vi "Teleop.vi"(10 "Match Info":T1={"Autonomous Elapsed Seconds"=0.0, "TeleOp Elapsed Seconds"=0.0, "Disabled Elapsed Seconds"=0.0, "Visited Autonomous"=FALSE, "Visited TeleOp"=FALSE, "Visited Disabled"=FALSE, "Autonomous Settings"={"Autonomous Style"=enum."Independent", "VI Refnum"=refnum}}, 11 "Call Context":T2) -> ()   [LabVIEW 2015]
doc: "This VI is called for each TeleOp packet received from the DS where the robot is not disabled. It is often used to read from the joysticks and update I/O or to update setpoints for timed control loops. It should complete and return within 20 milliseconds or it may miss DS packets."
uses:
  <vilib>/Rock Robotics/WPI/DriverStation/WPI_DriverStationDerivedRobotMode.ctl
  <vilib>/Rock Robotics/WPI/DriverStation/WPI_DriverStationMatch Info.ctl
  <vilib>/Rock Robotics/WPI/Solenoid/WPI_SolenoidValue.ctl
  <vilib>/Rock Robotics/Network Tables/NT Read Boolean.vi
  <vilib>/Rock Robotics/Network Tables/NT Read Number.vi
  <vilib>/Rock Robotics/WPI/Utilities/WPI_GetSetVariantRefNum.vi
  <vilib>/Rock Robotics/WPI/Solenoid/WPI_SolenoidSetEnum.vi
  <vilib>/addons/control/pid/pid.llb/PID (DBL).vi
  <vilib>/addons/control/pid/NI_PID_pid.lvlib
panel:
  in  "Numeric":dbl
  out "Encodeur gauche min":dbl
  out "Encodeur gauche max":dbl
  out "Encodeur droit max":dbl
  out "Encodeur droit min":dbl
  out "Sample Slider 0":dbl(slide) scale=0.0..5.0
  out "Sample Boolean 1":bool
  out "Sample Boolean 0":bool
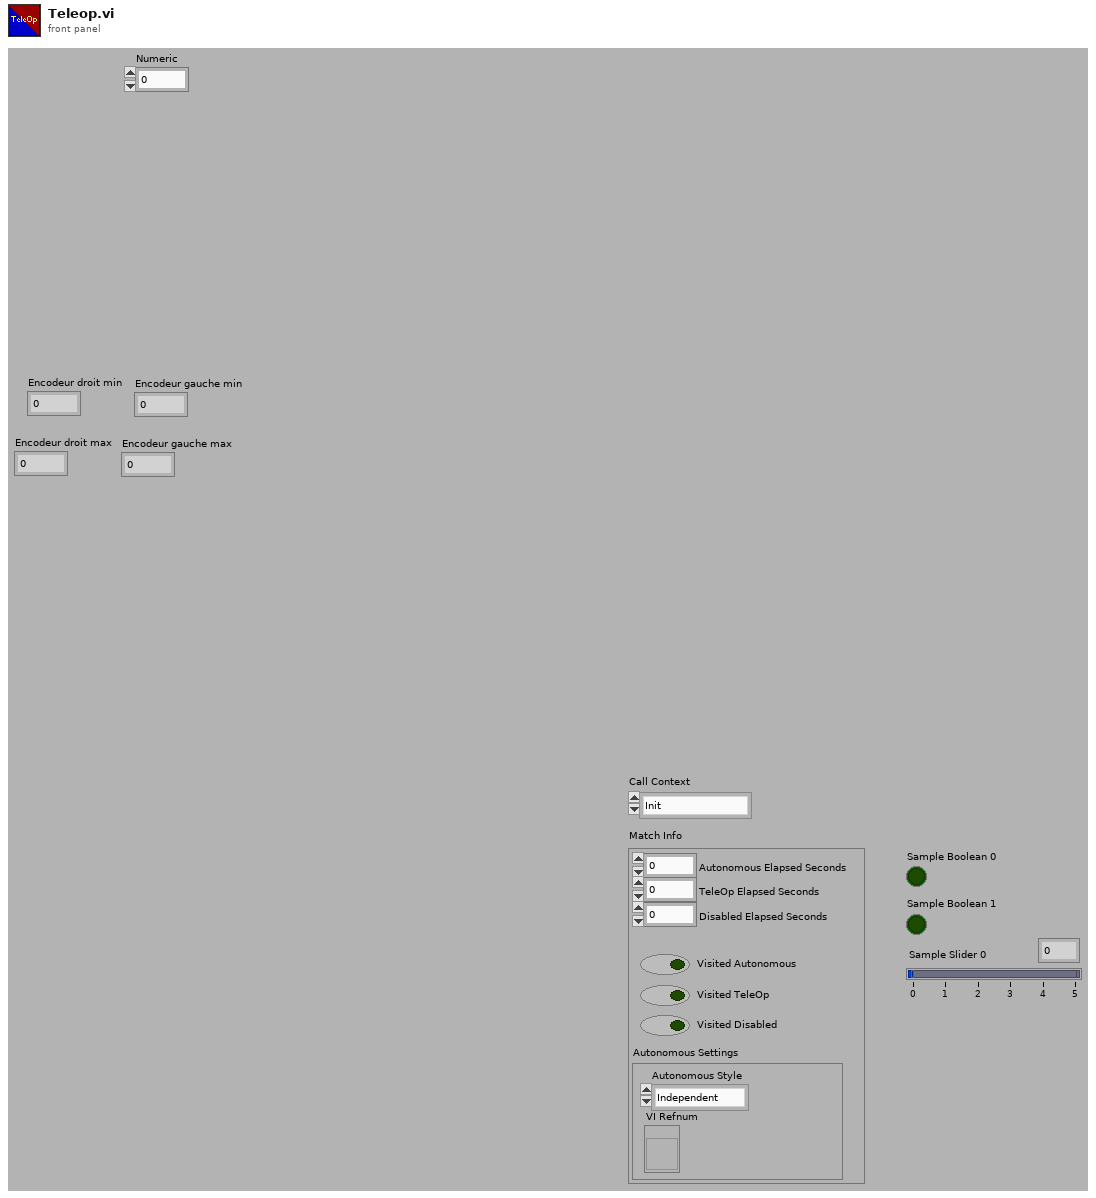
[diagram p1: front panel]
types:
  T1 = typedef "WPI_DriverStationMatch Info.ctl" = cluster{"Autonomous Elapsed Seconds":dbl, "TeleOp Elapsed Seconds":dbl, "Disabled Elapsed Seconds":dbl, "Visited Autonomous":bool, "Visited TeleOp":bool, "Visited Disabled":bool, "Autonomous Settings":cluster{"Autonomous Style":enum16{"Iterative", "Independent"}, "VI Refnum":refnum<vi>}}
  T2 = typedef "WPI_DriverStationDerivedRobotMode.ctl" = enum16{"Init", "Execute", "Stop"}
  T3 = typedef "WPI_JoystickDevRef.ctl" = cluster{"Device":T4}
  T4 = typedef "WPI_JoystickDeviceEnum.ctl" = enum16{"USB 0", "USB 1", "USB 2", "USB 3", "USB 4", "USB 5"}
  T5 = cluster{"Axes[0]":dbl, "Axes[1]":dbl, "Axes[2]":dbl, "Axes[3]":dbl, "Axes[4]":dbl, "Axes[5]":dbl, "Axes[6]":dbl, "Axes[7]":dbl, "Axes[8]":dbl}
  T6 = cluster{"Buttons[0]":bool, "Buttons[1]":bool, "Buttons[2]":bool, "Buttons[3]":bool, "Buttons[4]":bool, "Buttons[5]":bool, "Buttons[6]":bool, "Buttons[7]":bool, "Buttons[8]":bool}
  T7 = typedef "WPI_EncoderDevRef.ctl" = cluster{"DevStatus":errorcluster, "EncoderIndex":T8, "CounterIndex":T9, "DistancePerCount":dbl, "Decoding Type":T10}
  T8 = typedef "FPGA_EncoderIdx.ctl" = enum8{"Enc 0", "Enc 1", "Enc 2", "Enc 3", "Enc 4", "Enc 5", "Enc 6", "Enc 7", "Invalid"}
  T9 = typedef "FPGA_CounterCtrSystemIndex.ctl" = enum8{"Ctr 0", "Ctr 1", "Ctr 2", "Ctr 3", "Ctr 4", "Ctr 5", "Ctr 6", "Ctr 7", "Invalid"}
  T10 = typedef "WPI_EncoderType.ctl" = enum16{"1x", "2x", "4x"}
  T11 = cluster{"proportional gain (Kc)":dbl, "integral time (Ti, min)":dbl, "derivative time (Td, min)":dbl}
  T12 = typedef "WPI_SolenoidDevRef.ctl" = cluster{"DevStatus":errorcluster, "Pneumatics Control Module":u8, "Forward Solenoid Channel":T13, "Reverse Solenoid Channel":T13}
  T13 = typedef "WPI_SolenoidChannel.ctl" = enum8{"Solenoid 0", "Solenoid 1", "Solenoid 2", "Solenoid 3", "Solenoid 4", "Solenoid 5", "Solenoid 6", "Solenoid 7", "Invalid"}
  T14 = typedef "WPI_SolenoidValue.ctl" = enum16{"Off", "On", "Forward", "Reverse"}
  T15 = typedef "WPI_MotorControlDeviceRef.ctl" = cluster{"DeviceStatus":errorcluster, "Type":T16, "PWM":cluster{"PWM Channel":T17, "DeadBand":T18}, "CAN":cluster{"Device Number":u8, "Control Mode":T19, "Semaphore":T20, "Max Vout":dbl, "TalonSRX Control Mode":T21}, "Invert":bool}
  T16 = typedef "WPI_MotorControlType.ctl" = enum16{"PWM", "CAN", "CANTalonSRX"}
  T17 = typedef "FPGA_DIOPWMChannel.ctl" = enum8{"PWM 0", "PWM 1", "PWM 2", "PWM 3", "PWM 4", "PWM 5", "PWM 6", "PWM 7", "PWM 8", "PWM 9", "PWM MXP 0", "PWM MXP 1", "PWM MXP 2", "PWM MXP 3", "PWM MXP 4", "PWM MXP 5", "PWM MXP 6", "PWM MXP 7", "PWM MXP 8", "PWM MXP 9", "Invalid"}
  T18 = typedef "WPI_PWMDeadband.ctl" = cluster{"Name":string, "maxPositivePwm":i32, "minPositivePwm":i32, "centerPwm":i32, "maxNegativePwm":i32, "minNegativePwm":i32, "angularRange":u16}
  T19 = typedef "WPI_CANJaguar_ControlMode.ctl" = enum8{"Percent VBus", "Current", "Speed", "Position", "Voltage"}
  T20 = typedef "Semaphore RefNum" = refnum<k1>
  T21 = typedef "WPI_CANTalonSRX_APIControlMode.ctl" = enum8{"Percent VBus", "Speed", "Position", "Slave", "Unchanged / Invalid", "Voltage Compensation", "Current", "Motion Profile"}
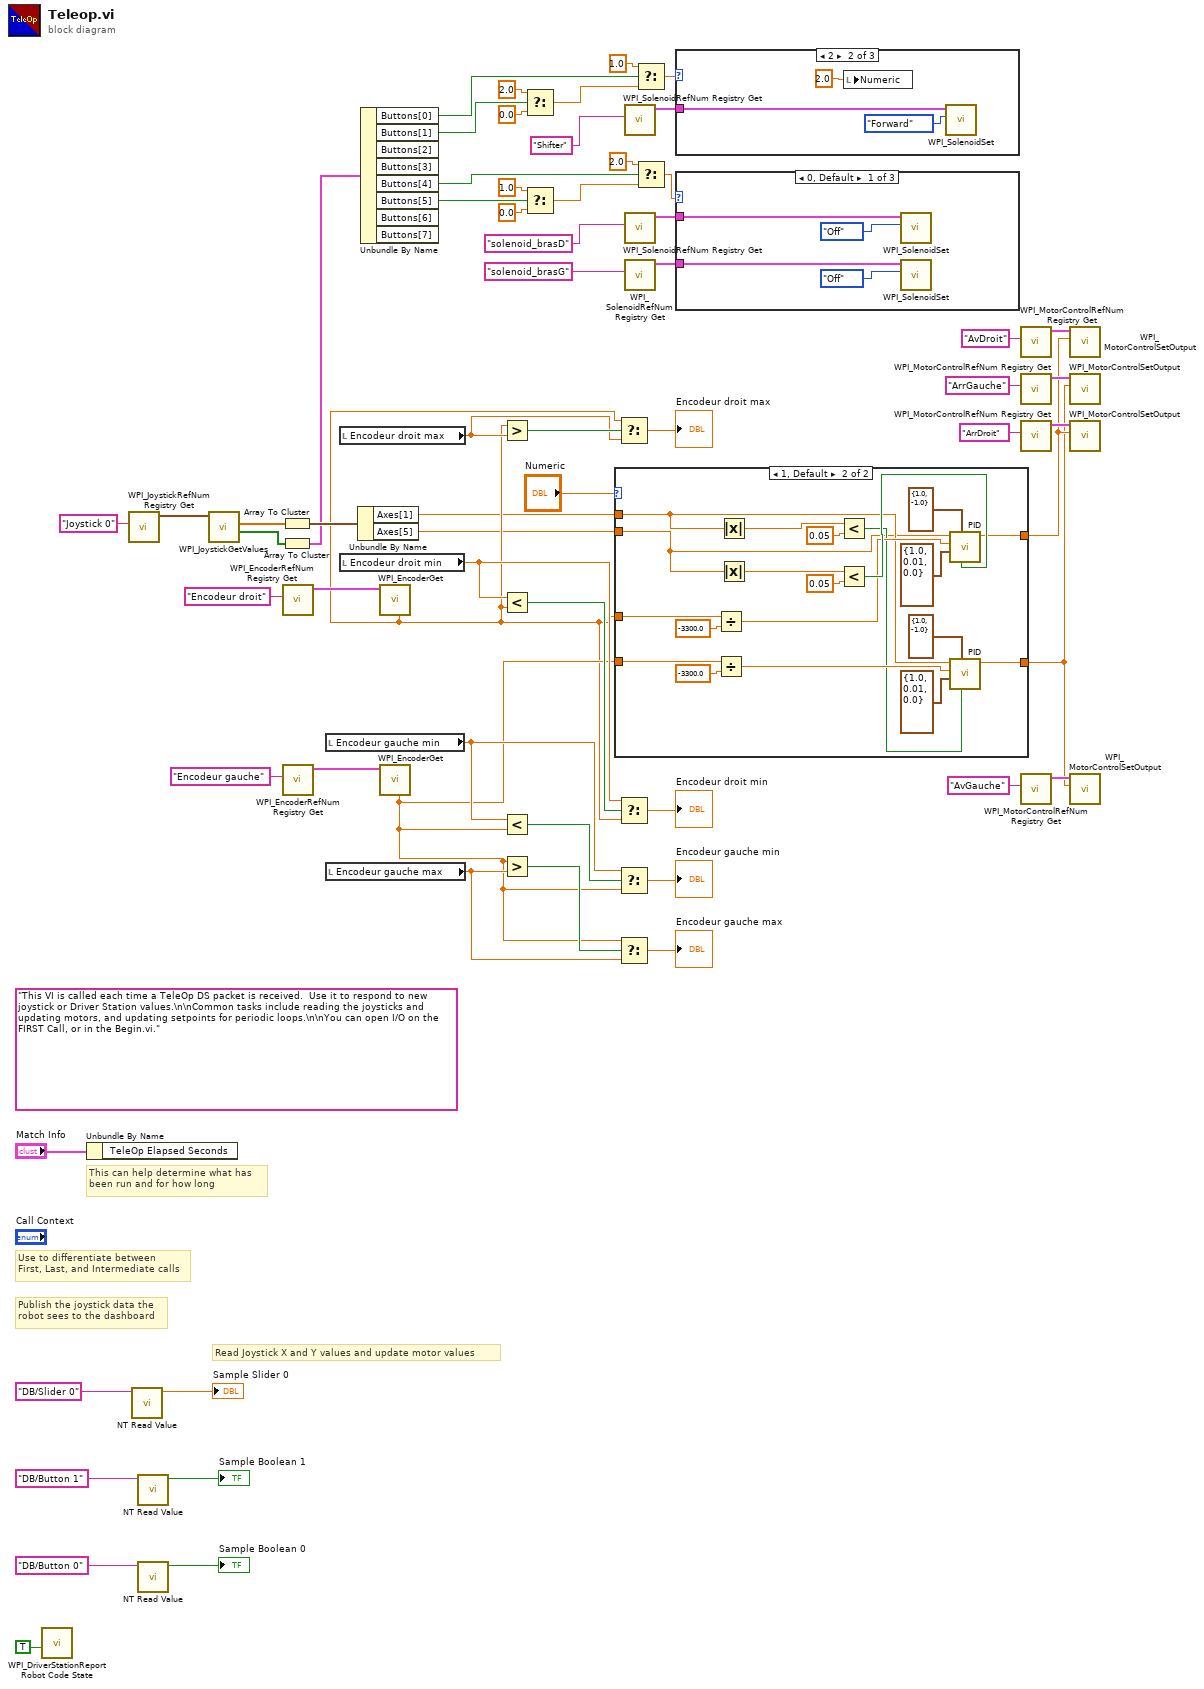
[diagram p0: block diagram]
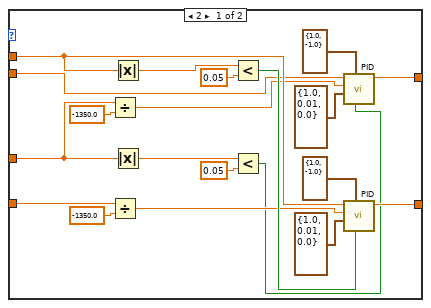
[diagram p2: hidden frame]
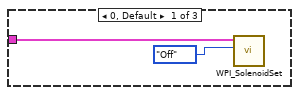
[diagram p3: hidden frame]
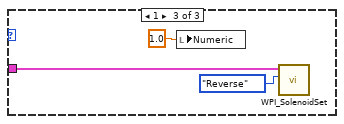
[diagram p4: hidden frame]
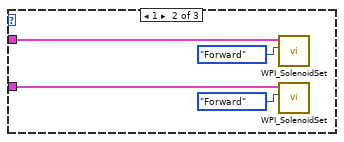
[diagram p5: hidden frame]
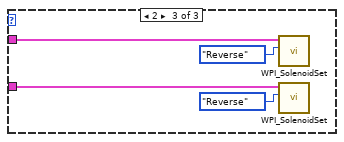
[diagram p6: hidden frame]
diagram:
  (unwired) "This VI is called each time a TeleOp DS packet is received.  Use it to respond to new joystick or Driver Station values.\n\nCommon tasks include reading the joysticks and updating motors, and updating setpoints for periodic loops.\n\nYou can open I/O on the FIRST Call, or in the Begin.vi."
  # "Publish the joystick data the\nrobot sees to the dashboard"
  # "Use to differentiate between\nFirst, Last, and Intermediate calls"
  # "This can help determine what has\nbeen run and for how long"
  # "Read Joystick X and Y values and update motor values"
  n1 = call <vilib>:"WPI_DriverStationReport Robot Code State.vi"("TeleOp"=TRUE ("Autonomous")) -> ()  [unwired: 10 in, 1 out]
  n2 = Unbundle By Name("Match Info") -> ()  [unwired: 1 out]
  n3 = call <vilib>:"WPI_JoystickRefNum Registry Get.vi"("refnum name"="Joystick 0") -> ("JoystickDevRef"=w56:T3)  [unwired: 1 in, 9 out]
  n4 = call-poly <vilib>:"NT Read Value.vi"("Name"="DB/Slider 0" ("refnum name")) -> ("Numeric"=→"Sample Slider 0":dbl)  [unwired: 9 in, 1 out]
  n5 = call-poly <vilib>:"NT Read Value.vi"("Name"="DB/Button 1" ("refnum name")) -> ("Boolean"=→"Sample Boolean 1":bool)  [unwired: 9 in, 1 out]
  n6 = call-poly <vilib>:"NT Read Value.vi"("Name"="DB/Button 0" ("refnum name")) -> ("Boolean"=→"Sample Boolean 0":bool)  [unwired: 9 in, 1 out]
  n7 = call <vilib>:"WPI_JoystickGetValues.vi"("JoystickDevRef"=w56) -> ("Buttons"=w53:bool[], "Axes"=w55:dbl[])  [unwired: 6 in, 3 out]
  n8 = Array To Cluster(array=w55) -> (cluster=w54:T5)
  n9 = Array To Cluster(array=w53) -> (cluster=w10:T6)
  n10 = call <vilib>:"WPI_EncoderRefNum Registry Get.vi"("refnum name"="Encodeur droit") -> ("EncoderDevRef"=w41:T7)  [unwired: 9 in, 1 out]
  n11 = call <vilib>:"WPI_EncoderRefNum Registry Get.vi"("refnum name"="Encodeur gauche") -> ("EncoderDevRef"=w40:T7)  [unwired: 9 in, 1 out]
  n12 = local read "Encodeur gauche min"() -> (w34:dbl)
  n13 = local read "Encodeur gauche max"() -> (w37:dbl)
  n14 = local read "Encodeur droit max"() -> (w32:dbl)
  n15 = local read "Encodeur droit min"() -> (w30:dbl)
  n16 = Unbundle By Name(w54) -> ("Axes[1]"=w3:dbl, "Axes[5]"=w5:dbl)
  n17 = Unbundle By Name(w10) -> ("Buttons[0]"=w9:bool, "Buttons[1]"=w8:bool, "Buttons[4]"=w7:bool, "Buttons[5]"=w6:bool)  [unwired: 4 out]
  n18 = call <vilib>:"WPI_EncoderGet.vi"("EncoderDevRef"=w41) -> ("Rate"=w18:dbl)  [unwired: 5 in, 5 out]
  n19 = call <vilib>:"WPI_EncoderGet.vi"("EncoderDevRef"=w40) -> ("Rate"=w19:dbl)  [unwired: 5 in, 5 out]
  n20 = Greater?(x=w18, y=w32) -> (0:w33:bool)
  n21 = Less?(x=w30, y=w18) -> (x < y?=w31:bool)
  n22 = Less?(x=w34, y=w19) -> (x < y?=w35:bool)
  n23 = Greater?(x=w19, y=w37) -> (0:w38:bool)
  n24 = Select(t=2.0, s=w8, f=0.0) -> (s? t:f=w50:dbl)
  n25 = Select(t=1.0, s=w6, f=0.0) -> (s? t:f=w48:dbl)
  n26 = case shown="1, Default" "Numeric" {
    tunnel: w3 -> [w77 w87]
    tunnel: [w78 w91] -> w2
    tunnel: w5 -> [w66 w86]
    tunnel: w18 -> [w67 w88]
    tunnel: [w69 w90] -> w4
    tunnel: w19 -> [w68 w89]
    frame 2 {
      n27 = Divide(x=w67, y=-1350.0) -> (x/y=w72:dbl)
      n28 = Divide(x=w68, y=-1350.0) -> (x/y=w81:dbl)
      n29 = Absolute Value(x=w77) -> (abs(x)=w83:dbl)
      n30 = Absolute Value(x=w67) -> (abs(x)=w74:dbl)
      n31 = Less?(x=w83, y=0.05) -> (x < y?=w85:bool)
      n32 = Less?(x=w74, y=0.05) -> (x < y?=w76:bool)
      n33 = call-poly <vilib>:"PID.vi"("reinitialize? (F)"=w76, "output range"=cluster{"output high":dbl, "output low":dbl} {"output high"=1.0, "output low"=-1.0}, "PID gains"=T11 {"proportional gain (Kc)"=1.0, "integral time (Ti, min)"=0.01, "derivative time (Td, min)"=0.0}, "process variable"=w72, "setpoint"=w66) -> ("output"=w69:dbl)  [unwired: 5 in, 1 out]
      n34 = call-poly <vilib>:"PID.vi"("reinitialize? (F)"=w85, "output range"=cluster{"output high":dbl, "output low":dbl} {"output high"=1.0, "output low"=-1.0}, "PID gains"=T11 {"proportional gain (Kc)"=1.0, "integral time (Ti, min)"=0.01, "derivative time (Td, min)"=0.0}, "process variable"=w81, "setpoint"=w77) -> ("output"=w78:dbl)  [unwired: 5 in, 1 out]
    }
    frame 1, Default {
      n35 = Divide(x=w88, y=-3300.0) -> (x/y=w95:dbl)
      n36 = Divide(x=w89, y=-3300.0) -> (x/y=w102:dbl)
      n37 = Absolute Value(x=w87) -> (abs(x)=w104:dbl)
      n38 = Absolute Value(x=w86) -> (abs(x)=w97:dbl)
      n39 = Less?(x=w104, y=0.05) -> (x < y?=w92:bool)
      n40 = Less?(x=w97, y=0.05) -> (x < y?=w99:bool)
      n41 = call-poly <vilib>:"PID.vi"("reinitialize? (F)"=w99, "output range"=cluster{"output high":dbl, "output low":dbl} {"output high"=1.0, "output low"=-1.0}, "PID gains"=T11 {"proportional gain (Kc)"=1.0, "integral time (Ti, min)"=0.01, "derivative time (Td, min)"=0.0}, "process variable"=w95, "setpoint"=w86) -> ("output"=w90:dbl)  [unwired: 5 in, 1 out]
      n42 = call-poly <vilib>:"PID.vi"("reinitialize? (F)"=w92, "output range"=cluster{"output high":dbl, "output low":dbl} {"output high"=1.0, "output low"=-1.0}, "PID gains"=T11 {"proportional gain (Kc)"=1.0, "integral time (Ti, min)"=0.01, "derivative time (Td, min)"=0.0}, "process variable"=w102, "setpoint"=w87) -> ("output"=w91:dbl)  [unwired: 5 in, 1 out]
    }
  }
  n43 = Select(t=w18, s=w33, f=w32) -> (s? t:f=→"Encodeur droit max":dbl)
  n44 = Select(t=w30, s=w31, f=w18) -> (s? t:f=→"Encodeur droit min":dbl)
  n45 = Select(t=w34, s=w35, f=w19) -> (s? t:f=→"Encodeur gauche min":dbl)
  n46 = Select(t=w19, s=w38, f=w37) -> (s? t:f=→"Encodeur gauche max":dbl)
  n47 = call <vilib>:"WPI_SolenoidRefNum Registry Get.vi"("refnum name"="Shifter") -> ("SolenoidDevRef"=w16:T12)  [unwired: 9 in, 1 out]
  n48 = call <vilib>:"WPI_SolenoidRefNum Registry Get.vi"("refnum name"="solenoid_brasD") -> ("SolenoidDevRef"=w11:T12)  [unwired: 9 in, 1 out]
  n49 = call <vilib>:"WPI_SolenoidRefNum Registry Get.vi"("refnum name"="solenoid_brasG") -> ("SolenoidDevRef"=w43:T12)  [unwired: 9 in, 1 out]
  n50 = Select(t=1.0, s=w9, f=w50) -> (s? t:f=w15:dbl)
  n51 = Select(t=2.0, s=w7, f=w48) -> (s? t:f=w44:dbl)
  n52 = case shown="2" w15 {
    tunnel: w16 -> [w107 w110 w112]
    frame 0, Default {
      n53 = call-poly <vilib>:"WPI_SolenoidSet.vi"("Value"=WPI_SolenoidValue."Off", "SolenoidDevRef"=w107) -> ()  [unwired: 8 in, 2 out]
    }
    frame 2 {
      n54 = local write "Numeric"(2.0 ("Numeric")) -> ()
      n55 = call-poly <vilib>:"WPI_SolenoidSet.vi"("Value"=WPI_SolenoidValue."Forward", "SolenoidDevRef"=w110) -> ()  [unwired: 8 in, 2 out]
    }
    frame 1 {
      n56 = local write "Numeric"(1.0 ("Numeric")) -> ()
      n57 = call-poly <vilib>:"WPI_SolenoidSet.vi"("Value"=WPI_SolenoidValue."Reverse", "SolenoidDevRef"=w112) -> ()  [unwired: 8 in, 2 out]
    }
  }
  n58 = case shown="0, Default" w44 {
    tunnel: w43 -> [w116 w121 w124]
    tunnel: w11 -> [w114 w118 w122]
    frame 0, Default {
      n59 = call-poly <vilib>:"WPI_SolenoidSet.vi"("Value"=WPI_SolenoidValue."Off", "SolenoidDevRef"=w114) -> ()  [unwired: 8 in, 2 out]
      n60 = call-poly <vilib>:"WPI_SolenoidSet.vi"("Value"=WPI_SolenoidValue."Off", "SolenoidDevRef"=w116) -> ()  [unwired: 8 in, 2 out]
    }
    frame 1 {
      n61 = call-poly <vilib>:"WPI_SolenoidSet.vi"("Value"=WPI_SolenoidValue."Forward", "SolenoidDevRef"=w118) -> ()  [unwired: 8 in, 2 out]
      n62 = call-poly <vilib>:"WPI_SolenoidSet.vi"("Value"=WPI_SolenoidValue."Forward", "SolenoidDevRef"=w121) -> ()  [unwired: 8 in, 2 out]
    }
    frame 2 {
      n63 = call-poly <vilib>:"WPI_SolenoidSet.vi"("Value"=WPI_SolenoidValue."Reverse", "SolenoidDevRef"=w122) -> ()  [unwired: 8 in, 2 out]
      n64 = call-poly <vilib>:"WPI_SolenoidSet.vi"("Value"=WPI_SolenoidValue."Reverse", "SolenoidDevRef"=w124) -> ()  [unwired: 8 in, 2 out]
    }
  }
  n65 = call <vilib>:"WPI_MotorControlRefNum Registry Get.vi"("refnum name"="AvDroit") -> ("MotorControlDevRef"=w25:T15)  [unwired: 9 in, 1 out]
  n66 = call <vilib>:"WPI_MotorControlRefNum Registry Get.vi"("refnum name"="ArrGauche") -> ("MotorControlDevRef"=w26:T15)  [unwired: 9 in, 1 out]
  n67 = call <vilib>:"WPI_MotorControlRefNum Registry Get.vi"("refnum name"="ArrDroit") -> ("MotorControlDevRef"=w24:T15)  [unwired: 9 in, 1 out]
  n68 = call <vilib>:"WPI_MotorControlRefNum Registry Get.vi"("refnum name"="AvGauche") -> ("MotorControlDevRef"=w27:T15)  [unwired: 9 in, 1 out]
  n69 = call <vilib>:"WPI_MotorControlSetOutput.vi"("Output"=w4, "MotorControlDevRef"=w25) -> ()  [unwired: 7 in, 3 out]
  n70 = call <vilib>:"WPI_MotorControlSetOutput.vi"("Output"=w2, "MotorControlDevRef"=w26) -> ()  [unwired: 7 in, 3 out]
  n71 = call <vilib>:"WPI_MotorControlSetOutput.vi"("Output"=w4, "MotorControlDevRef"=w24) -> ()  [unwired: 7 in, 3 out]
  n72 = call <vilib>:"WPI_MotorControlSetOutput.vi"("Output"=w2, "MotorControlDevRef"=w27) -> ()  [unwired: 7 in, 3 out]
